vi "Filter Get Averaging Factor.vi"(8 "error in (no error)":errorcluster, 11 "averagingFactor":i32) -> (0 "error out":errorcluster, 2 "function return":u32, 3 "averagingFactor out":i32)   [LabVIEW 2014, in "atmcd32d.lvlib"]
doc: "unsigned int WINAPI Filter_GetAveragingFactor(int * averagingFactor);"
uses:
  atmcd32d.lvlib
  atmcd32d.dll
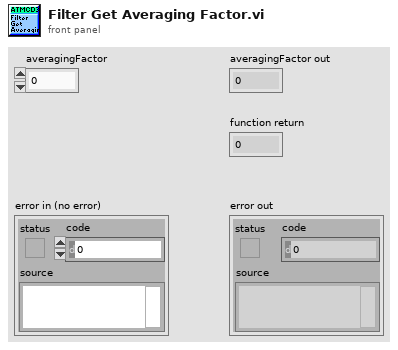
[diagram p1: front panel]
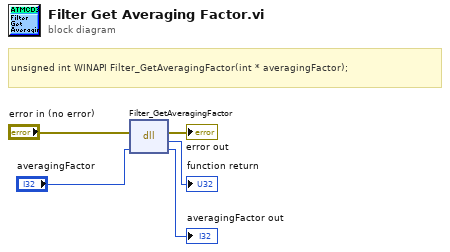
[diagram p0: block diagram]
diagram:
  # "unsigned int WINAPI Filter_GetAveragingFactor(int * averagingFactor);"
  n1 = dll-call lib="C:/Users/Bakir/Documents/Lambda2-Testing/lib/Andorlib/atmcd32d.*" fn="Filter_GetAveragingFactor"(error in="error in (no error)", "averagingFactor"="averagingFactor") -> (error out=→"error out":errorcluster, →"function return":u32, "averagingFactor"=→"averagingFactor out":i32)  [unwired: 2 in, 1 out]
